vi "Main Engine Check and Delete Backup File.vi"(8 "error in":errorcluster) -> (0 "error out":errorcluster, 3 "Data File Path":path)   [LabVIEW 2018]
doc: "All Rights Reserved © 2023 SyncSols"
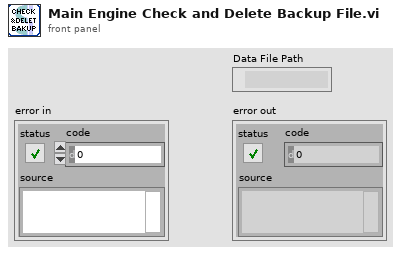
[diagram p1: front panel]
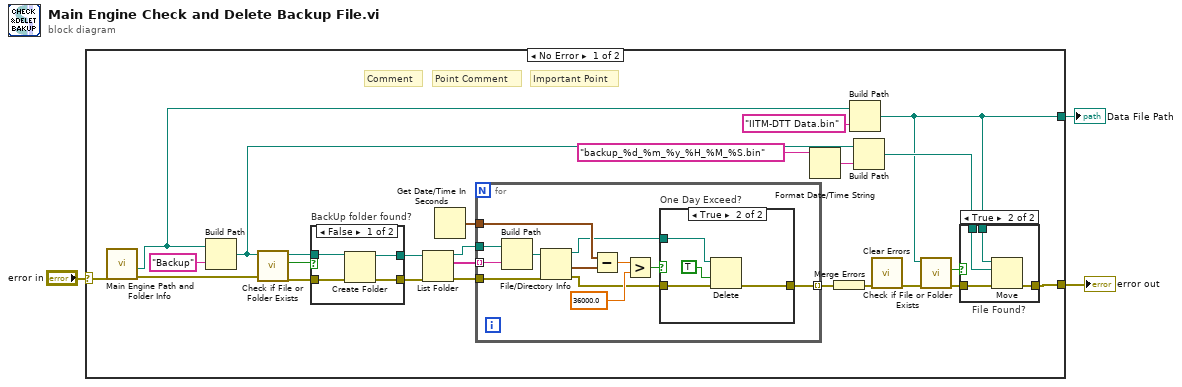
[diagram p0: block diagram]
diagram:
  n1 = case shown="No Error" "error in" {
    selector: "error in" -> [w5 w57]
    tunnel: [w8 w57] -> w3
    tunnel: [w7 _] -> w1
    frame No Error {
      # "Important Point"
      # "Point Comment"
      # "Comment"
      n2 = call "Main Engine Path and Folder Info.vi"("error in"=w5) -> ("error out"=w4:errorcluster, "LabVIEW Data"=w6:path)  [unwired: 5 in, 4 out]
      n3 = Build Path(base path=w6, name or relative path="Backup") -> (appended path=w15:path)
      n4 = call <vilib>:"Check if File or Folder Exists.vi"("error in (no error)"=w4, "path"=w15) -> ("error out"=w25:errorcluster, "file or folder exists?"=w27:bool, "dup path"=w26:path)  [unwired: 7 in]
      n5 = case "BackUp folder found?" shown="False" w27 {
        tunnel: w26 -> [w54 w56]
        tunnel: w25 -> [w53 w55]
        tunnel: [w52 w56] -> w23
        tunnel: [w51 w55] -> w24
        frame False {
          n6 = Create Folder(path (use dialog)=w54, error in=w53) -> (created path=w52:path, error out=w51:errorcluster)  [unwired: 1 in, 1 out]
        }
        frame True {
        }
      }
      n7 = List Folder(path=w23, error in=w24) -> (path out=w21:path, filenames=w20:string[], error out=w22:errorcluster)  [unwired: 2 in, 1 out]
      n8 = Get Date/Time In Seconds() -> (seconds since 1Jan1904=w19:timestamp)
      n9 = for {
        tunnel: w22 -> [w42]
        tunnel: w21 -> [w44]
        tunnel: w20 -> [w45] mode=indexing
        tunnel: w19 -> [w41]
        tunnel: [w34] -> w18 mode=indexing
        n10 = Build Path(base path=w44, name or relative path=w45) -> (appended path=w43:path)
        n11 = File/Directory Info(path=w43, error in=w42) -> (path out=w36:path, last mod=w40:timestamp, error out=w35:errorcluster)  [unwired: 4 out]
        n12 = Subtract(x=w41, y=w40) -> (x-y=w39:dbl)
        n13 = Greater?(x=w39, y=36000.0) -> (0:w37:bool)
        n14 = case "One Day Exceed?" shown="True" w37 {
          tunnel: w36 -> [_ w50]
          tunnel: w35 -> [w46 w48]
          tunnel: [w46 w47] -> w34
          frame False {
          }
          frame True {
            n15 = Delete(path (use dialog)=w50, confirm (F)=TRUE, error in=w48) -> (error out=w47:errorcluster)  [unwired: 2 in, 2 out]
          }
        }
      }
      n16 = Format Date/Time String(time format string (%c)="backup_%d_%m_%y_%H_%M_%S.bin") -> (date/time string=w14:string)  [unwired: 2 in]
      n17 = Merge Errors(w18) -> (w16:errorcluster)
      n18 = Build Path(base path=w6, name or relative path="IITM-DTT Data.bin") -> (appended path=w7:path)
      n19 = Build Path(base path=w15, name or relative path=w14) -> (appended path=w12:path)
      n20 = call <vilib>:"Clear Errors.vi"("error in (no error)"=w16) -> ("error out"=w11:errorcluster)  [unwired: 5 in, 1 out]
      n21 = call <vilib>:"Check if File or Folder Exists.vi"("error in (no error)"=w11, "path"=w7) -> ("error out"=w10:errorcluster, "file or folder exists?"=w9:bool)  [unwired: 7 in, 1 out]
      n22 = case "File Found?" shown="True" w9 {
        tunnel: w12 -> [_ w33]
        tunnel: w10 -> [w29 w32]
        tunnel: w7 -> [_ w31]
        tunnel: [w29 w30] -> w8
        frame False {
        }
        frame True {
          n23 = Move(source path=w31, error in=w32, 10:w33) -> (error out=w30:errorcluster)  [unwired: 2 in, 2 out]
        }
      }
    }
    frame Error {
    }
  }
  "error out" <- w3
  "Data File Path" <- w1
